vi "Client Connect To IP Test.vi"() -> ()   [LabVIEW 2014, in "ESP8266 WiFi Wrapper.lvlib"]
uses:
  ESP8266 WiFi Wrapper.lvlib
panel:
  out "Connected?":bool
  in  "Port":u32=8080
  in  "IP address":u8[](array[numeric])=[127, 0, 0, 1]
  out "Error Out":errorcluster
  in  "Error In":errorcluster
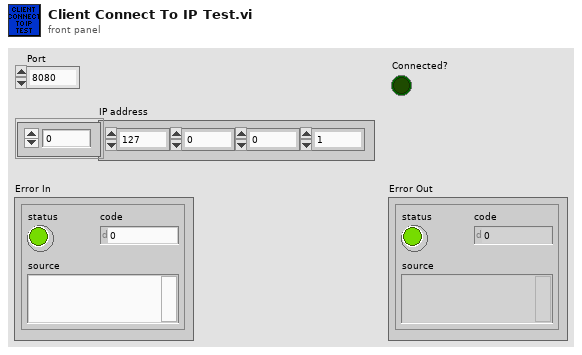
[diagram p1: front panel]
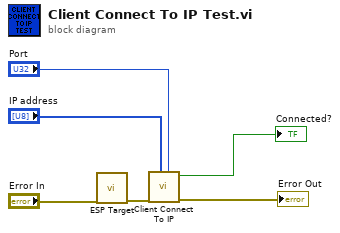
[diagram p0: block diagram]
diagram:
  n1 = call "ESP Target.vi"("Error In"="Error In") -> ("Error Out"=w1:errorcluster)  [unwired: 10 in]
  n2 = call "Client Connect To IP.vi"("Port"="Port", "IP address"="IP address", "Error In"=w1) -> ("Error Out"=→"Error Out":errorcluster, "Connected?"=→"Connected?":bool)  [unwired: 7 in]
